vi "TRA speed.vi"(9 "t2":dbl format="%#_13g", 10 "i":i32, 11 "dt(s)":dbl) -> (0 "complet?":bool, 3 "Waveform Chart":dbl(graph))   [LabVIEW 2019]
panel:
  out "second":dbl
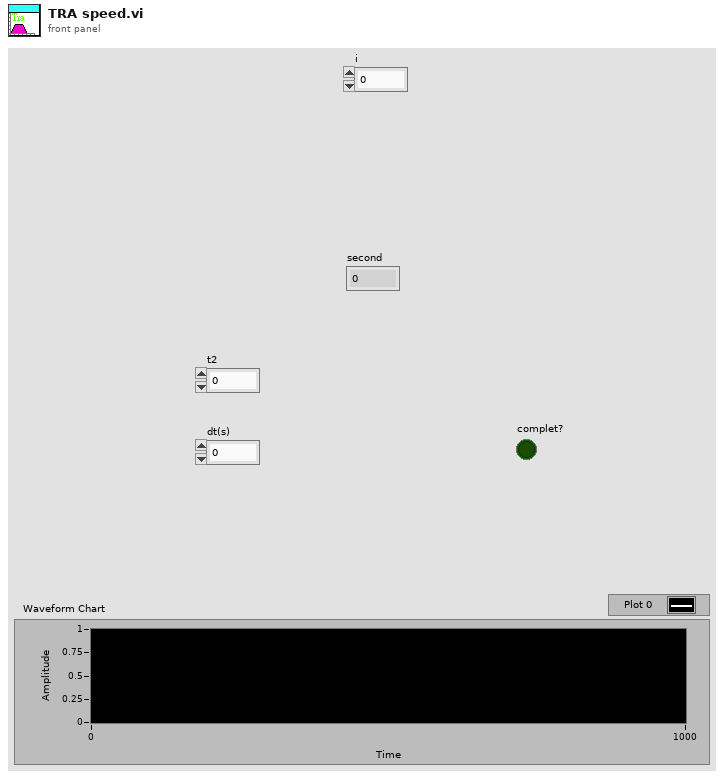
[diagram p1: front panel]
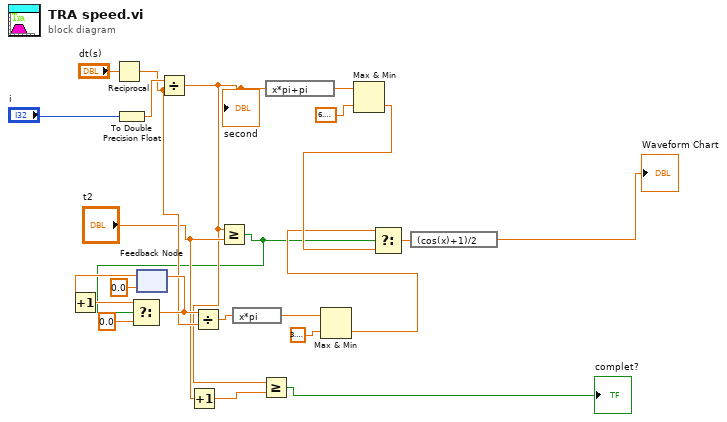
[diagram p0: block diagram]
diagram:
  n1 = Reciprocal(x="dt(s)") -> (1/x=w12:dbl)
  n2 = To Double Precision Float(number="i") -> (double precision float=w22:dbl)
  n3 = feedback #1(0.0 ("f")) -> (w16:dbl)
  n4 = Increment(x=w16) -> (x+1=w14:dbl)
  n5 = Divide(x=w22, y=w12) -> (x/y=w4:dbl)
  "second" <- w4
  n6 = Increment(x="t2") -> (x+1=w5:dbl)
  n7 = Greater Or Equal?(x=w4, y="t2") -> (x >= y?=w3:bool)
  n8 = Select(t=w14, s=w3, f=0.0) -> (s? t:f=w13:dbl)
  n9 = feedback-in #1(w13) -> ()
  n10 = Divide(x=w13, y=w12) -> (x/y=w11:dbl)
  n11 = expression code="x*pi"(w11) -> (w10:dbl)
  n12 = Greater Or Equal?(x=w4, y=w5) -> (x >= y?=→"complet?":bool)
  n13 = expression code="x*pi+pi"(w4) -> (w21:dbl)
  n14 = Max & Min(x=w10, y=3.141592653589793) -> (min(x,y)=w8:dbl)  [unwired: 1 out]
  n15 = Max & Min(x=w21, y=6.283185307179586) -> (min(x,y)=w19:dbl)  [unwired: 1 out]
  n16 = Select(t=w8, s=w3, f=w19) -> (s? t:f=w18:dbl)
  n17 = expression code="(cos(x)+1)/2"(w18) -> (→"Waveform Chart":dbl)
